vi "XY to Linear Address (SubVI).vi"(1 "X":u16, 2 "Y":u16, 3 "Image Width":u16) -> (4 "Linear Address":u32)   [LabVIEW 2015]
uses:
  <vilib>/rvi/FXPMathLib/FxpMul/XNode/nifxpmath_Multiplier.xnode
  <vilib>/rvi/FXPMathLib/FxpAdd/XNode/nifxpmath_Add.xnode
  <vilib>/rvi/FXPMathLib/sim/FxpSim.dll
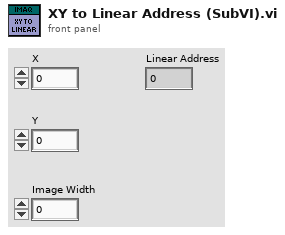
[diagram p1: front panel]
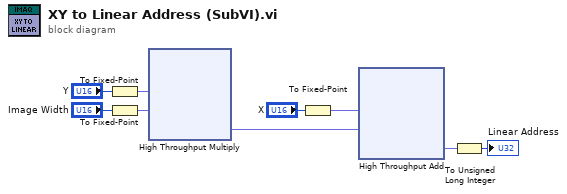
[diagram p0: block diagram]
diagram:
  n1 = To Fixed-Point(number="Y") -> (fixed-point=w7:fxp<+,12,12>)  [unwired: 1 in]
  n2 = To Fixed-Point(number="Image Width") -> (fixed-point=w8:fxp<+,12,12>)  [unwired: 1 in]
  n3 = xnode ("High Throughput Multiply")("x"=w7, "y"=w8) -> ("x*y"=w3:fxp<+,24,24>)
  n4 = To Fixed-Point(number="X") -> (fixed-point=w4:fxp<+,12,12>)  [unwired: 1 in]
  n5 = xnode ("High Throughput Add")("x"=w4, "y"=w3) -> ("x+y"=w2:fxp<+,24,24>)
  n6 = To Unsigned Long Integer(number=w2) -> (unsigned 32bit integer=→"Linear Address":u32)
